vi "FieldDisp_Field_Crop_and_Scale.vi"(4 "Field Y Ft":dbl=27.0 format="%#_13g", 5 "Disp Y Size Pixel":i32=-1, 6 "Field X Ft":dbl=58.0 format="%#_13g", 7 "Disp X Size Pixel":i32=-1, 9 "Field Image":T1, 10 "field Info":T2, 11 "Field Picture Ref":refnum<vi>) -> (0 "error out":errorcluster)   [LabVIEW 2019, in "Trajectory_Library.lvlib"]
doc: "Internal function -- should not be called directly by users.\n\nComplete documentation TBD."
uses:
  Trajectory_Library.lvlib
  TypeDef/FieldDisp_Field_Info.ctl
  <vilib>/vision/Image Controls.llb/IMAQ Image.ctl
  <vilib>/Utility/miscctls.llb/LVBoundsTypeDef.ctl
  <vilib>/vision/NI_Vision_Development_Module.lvlib
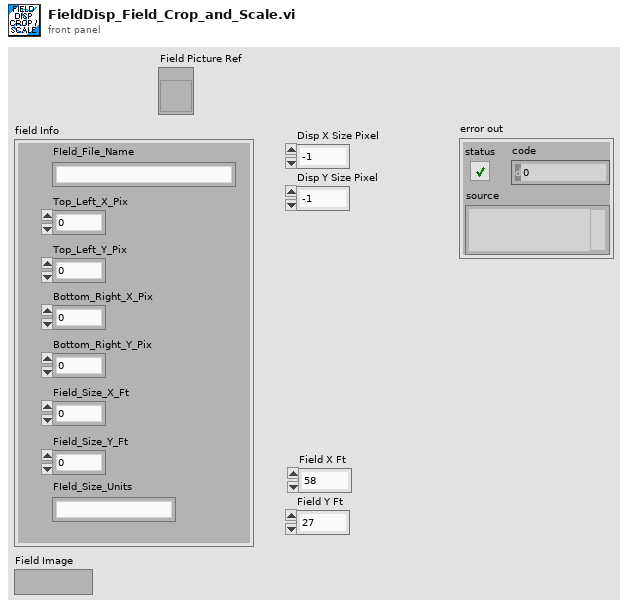
[diagram p1: front panel]
types:
  T1 = typedef "IMAQ Image.ctl" = refnum<image>
  T2 = typedef "Trajectory_Library.lvlib/FieldDisp_Field_Info.ctl" = cluster{"FIeld_File_Name":string, "Top_Left_X_Pix":i32, "Top_Left_Y_Pix":i32, "Bottom_Right_X_Pix":i32, "Bottom_Right_Y_Pix":i32, "Field_Size_X_Ft":dbl, "Field_Size_Y_Ft":dbl, "FIeld_Size_Units":string}
  T3 = typedef "Image Type" = u32
  T4 = typedef "LVBoundsTypeDef.ctl" = cluster{"Width":u32, "Height":u32}
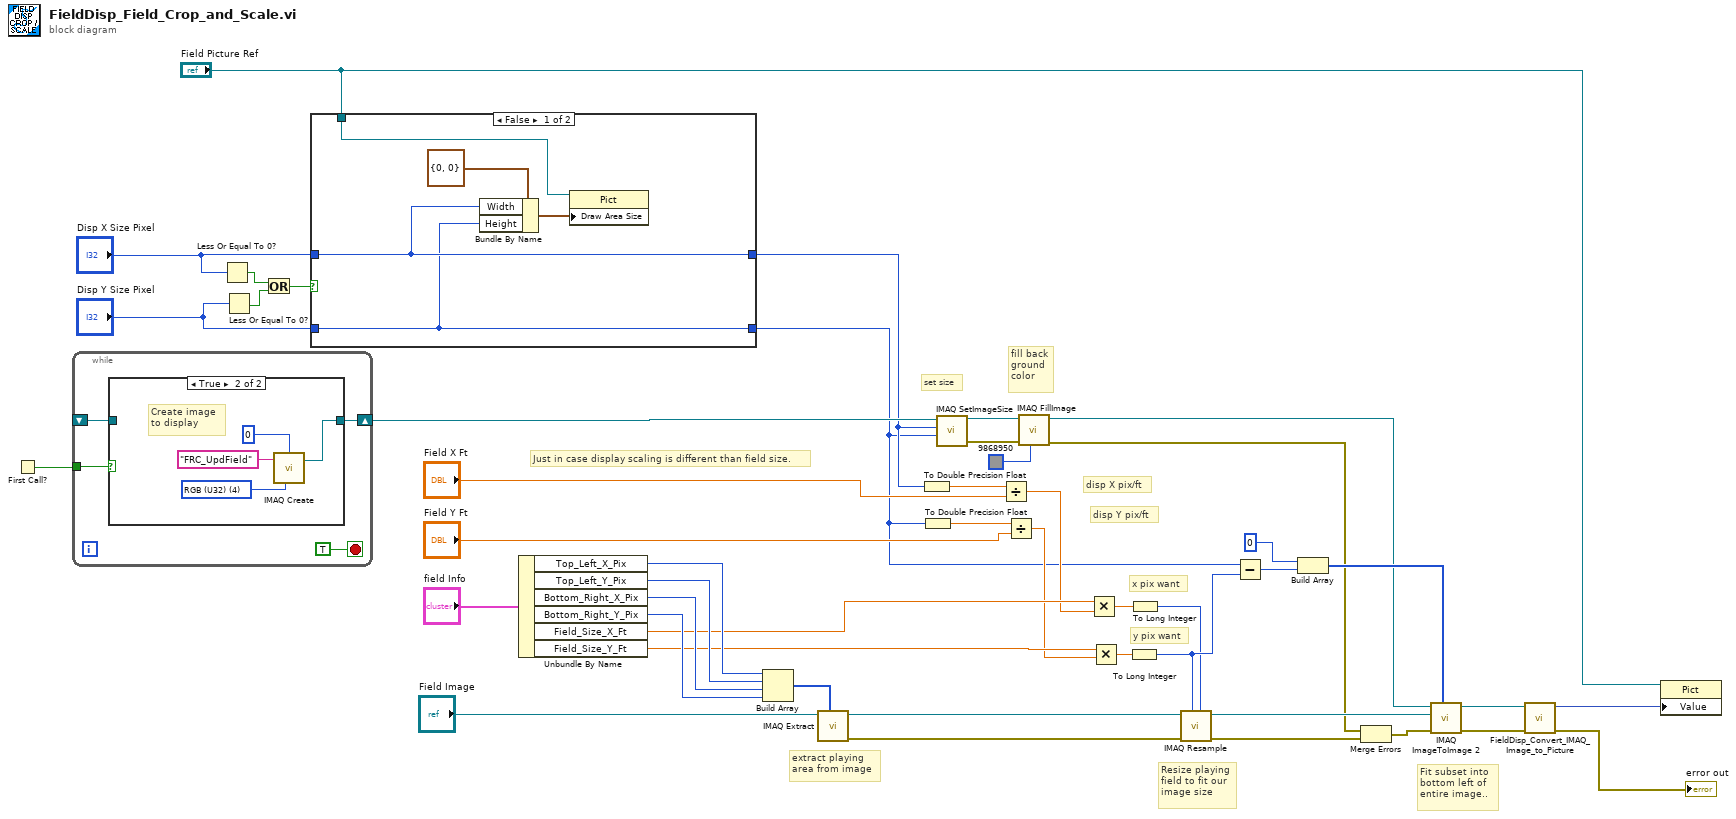
[diagram p0: block diagram]
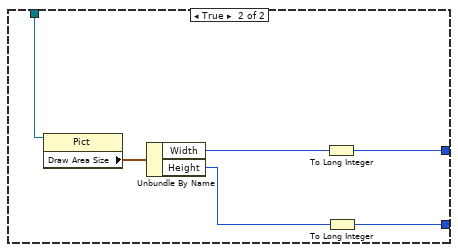
[diagram p2: hidden frame]
diagram:
  # "Just in case display scaling is different than field size."
  # "Resize playing\nfield to fit our\nimage size"
  # "disp Y pix/ft"
  # "extract playing \narea from image"
  # "y pix want"
  # "x pix want"
  # "disp X pix/ft"
  # "fill back\nground\ncolor"
  # "set size"
  # "Fit subset into\nbottom left of \nentire image.."
  n1 = First Call?() -> (First Call?: T/F=w18:bool)
  n2 = while {
    tunnel: w18 -> [w49]
    shift-right: [w48] -> w17
    shift-left: _ -> [w47]
    stop <- TRUE stop-if-true
    n3 = case shown="True" w49 {
      tunnel: [w51 w52] -> w48
      tunnel: w47 -> [w51 _]
      frame False {
      }
      frame True {
        w53 = T3 4 items=["Grayscale (U8)", "Grayscale (I16)", "Grayscale (SGL)", "Complex (CSG)", "RGB (U32)", "HSL (U32)", "RGB (U64)", "Grayscale (U16)"] ("Image Type")
        # "Create image \nto display"
        n4 = call "IMAQ Create"("Border Size"=0, "Image Name"="FRC_UpdField", "Image Type"=w53) -> ("New Image"=w52:T1)  [unwired: 2 in, 1 out]
      }
    }
  }
  n5 = Less Or Equal To 0?(x="Disp X Size Pixel") -> (x <= 0?=w12:bool)
  n6 = Less Or Equal To 0?(x="Disp Y Size Pixel") -> (x <= 0?=w11:bool)
  n7 = Or(x=w12, y=w11) -> (x .or. y?=w10:bool)
  n8 = case shown="False" w10 {
    tunnel: "Disp X Size Pixel" -> [w58 _]
    tunnel: [w58 w61] -> w15
    tunnel: "Disp Y Size Pixel" -> [w57 _]
    tunnel: [w57 w63] -> w13
    tunnel: "Field Picture Ref" -> [w56 w66]
    frame False {
      n9 = Bundle By Name(cluster=T4 {"Width"=0, "Height"=0} ("Draw Area Size"), "Width"=w58, "Height"=w57) -> (w60:T4)
      n10 = property on="Property Node" class="Pict"(reference=w56, "Draw Area Size"=w60) -> ()  [unwired: 1 in, 2 out]
    }
    frame True {
      n11 = property on="Property Node" class="Pict"(reference=w66) -> ("Draw Area Size"=w65:T4)  [unwired: 1 in, 2 out]
      n12 = Unbundle By Name(w65) -> ("Width"=w62:u32, "Height"=w64:u32)
      n13 = To Long Integer(number=w62) -> (32bit integer=w61:i32)
      n14 = To Long Integer(number=w64) -> (32bit integer=w63:i32)
    }
  }
  n15 = Unbundle By Name("field Info") -> ("Top_Left_X_Pix"=w43:i32, "Top_Left_Y_Pix"=w44:i32, "Bottom_Right_X_Pix"=w45:i32, "Bottom_Right_Y_Pix"=w46:i32, "Field_Size_X_Ft"=w39:dbl, "Field_Size_Y_Ft"=w40:dbl)
  n16 = Build Array(w43, w44, w45, w46) -> (w21:i32[])
  n17 = call "IMAQ Extract"("Optional Rectangle"=w21, "Image Src"="Field Image") -> ("error out"=w6:errorcluster, "Image Dst Out"=w30:T1)  [unwired: 8 in]
  n18 = To Double Precision Float(number=w15) -> (double precision float=w24:dbl)
  n19 = To Double Precision Float(number=w13) -> (double precision float=w25:dbl)
  n20 = call "IMAQ SetImageSize"("Y Resolution"=w13, "X Resolution"=w15, "Image"=w17) -> ("error out"=w7:errorcluster, "Image Out"=w22:T1)  [unwired: 2 in]
  n21 = Divide(x=w24, y="Field X Ft") -> (x/y=w28:dbl)
  n22 = Divide(x=w25, y="Field Y Ft") -> (x/y=w29:dbl)
  n23 = call "IMAQ FillImage"("Color Pixel Value"=u32 9868950, "error in (no error)"=w7, "Image"=w22) -> ("error out"=w4:errorcluster, "Image Out"=w34:T1)  [unwired: 7 in]
  n24 = Multiply(x=w39, y=w28) -> (x*y=w32:dbl)
  n25 = Multiply(x=w40, y=w29) -> (x*y=w33:dbl)
  n26 = To Long Integer(number=w33) -> (32bit integer=w36:i32)
  n27 = To Long Integer(number=w32) -> (32bit integer=w31:i32)
  n28 = call "IMAQ Resample"("X Resolution"=w31, "Y Resolution"=w36, "error in (no error)"=w6, "Image Src"=w30) -> ("error out"=w3:errorcluster, "Image Dst Out"=w37:T1)  [unwired: 6 in]
  n29 = Subtract(x=w13, y=w36) -> (x-y=w41:i32)
  n30 = Build Array(0, w41) -> (w38:i32[])
  n31 = Merge Errors(w4, w3) -> (w5:errorcluster)
  n32 = call "IMAQ ImageToImage 2"("Offset Left/Top"=w38, "error in (no error)"=w5, "Image Src (Small)"=w37, "Image Src (Large)"=w34) -> ("error out"=w2:errorcluster, "Image Dst Out"=w19:T1)  [unwired: 6 in]
  n33 = call "FieldDisp_Convert_IMAQ_Image_to_Picture.vi"("error in (no error)"=w2, "Image In"=w19) -> ("error out"=→"error out":errorcluster, "new picture"=w9:picture)  [unwired: 8 in]
  n34 = property on="Property Node" class="Pict"(reference="Field Picture Ref", "Value"=w9) -> ()  [unwired: 1 in, 2 out]
